vi "ClusterEscala.vi"() -> ()   [LabVIEW 2020]
panel:
  out "Cluster 2":T1 {"Slide" scale=0.0..100.0; "Gauge" scale=0.0..40.0; "Thermometer" scale=0.0..50.0}
  out "x*y":cluster{dbl, dbl, dbl}
  in  "Cluster":T2
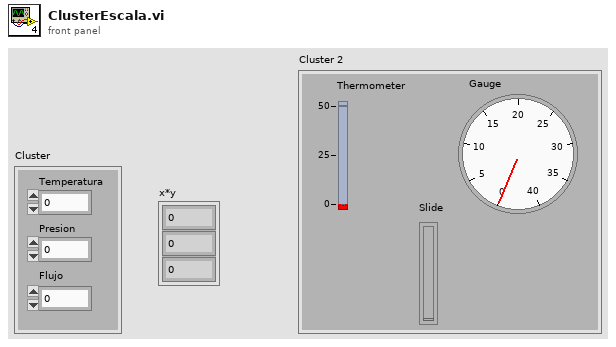
[diagram p1: front panel]
types:
  T1 = cluster{"Thermometer":dbl, "Gauge":dbl, "Slide":u8}
  T2 = cluster{"Temperatura":dbl, "Presion":dbl, "Flujo":dbl}
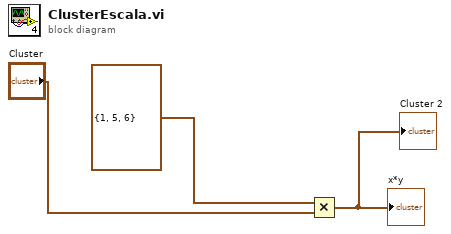
[diagram p0: block diagram]
diagram:
  n1 = Multiply(x=cluster{i32, i32, i32} {1, 5, 6}, y="Cluster") -> (x*y=→"x*y" →"Cluster 2":cluster{dbl, dbl, dbl})
